vi "Read HK DVR.vi"(8 "error in (no error)":errorcluster, 11 "eCRDS in":refnum<class "eCRDS.lvclass">) -> (0 "error out":errorcluster, 2 "HK DVR":refnum<data-value>, 3 "eCRDS out":refnum<class "eCRDS.lvclass">)   [LabVIEW 2014, in "eCRDS.lvclass"]
uses:
  eCRDS.lvclass
  eCRDS.lvclass/eCRDS.ctl
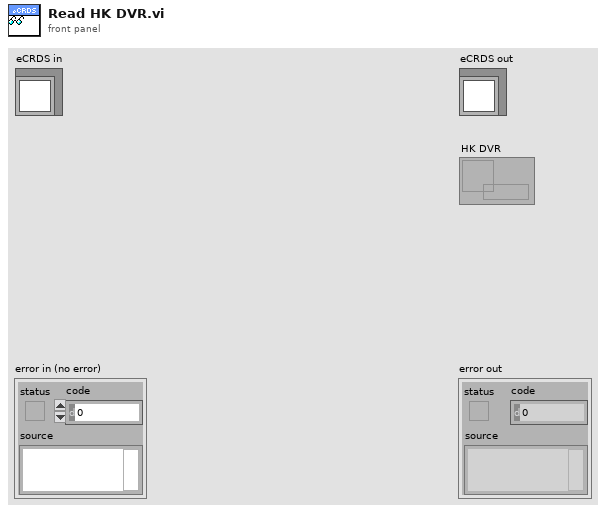
[diagram p1: front panel]
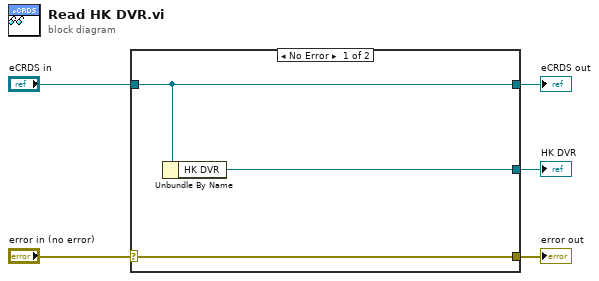
[diagram p0: block diagram]
diagram:
  n1 = case shown="No Error" "error in (no error)" {
    selector: "error in (no error)" -> [w8 w9]
    tunnel: [w8 w9] -> w4
    tunnel: [w7 w10] -> w2
    tunnel: "eCRDS in" -> [w7 w10]
    tunnel: [w6 _] -> w1
    frame No Error {
      n2 = Unbundle By Name(w7) -> ("HK DVR"=w6:refnum<data-value>)
    }
    frame Error {
    }
  }
  "error out" <- w4
  "eCRDS out" <- w2
  "HK DVR" <- w1
